vi "MirrorSlide2xPan.vi"(8 "error in (no error)":errorcluster caption="entrée d'erreur (pas d'erreur)", 11 "ESP301.lvclass":refnum<class "ESP301.lvclass">) -> (0 "error out":errorcluster caption="sortie d'erreur", 3 "ESP301.lvclass Out":refnum<class "ESP301.lvclass">)   [LabVIEW 2019, in "ESP301.lvclass"]
uses:
  ESP301.lvclass
  C:/Programmes Labview/LabScanV1A/DevicesClass/BaseDevice/BaseDevice.lvclass
  ESP301.lvclass/ESP301.ctl
  BaseDevice/ClassQueueMess.ctl
  BaseDevice/Accessor/GetClassEvent.vi
panel:
  out "ActPos 2":dbl=60.0 caption="Pos(mm)" min=0.1 step=0.1 format="%#.4f"
  in  "Motion ax2":u16(ring) caption="MiseAJour" items=["Cam", "APD", "Spectro"]
  out "Mvg_ax2":bool caption="Moving"
  out "Hmd_ax2":bool caption="Homed"
  in  "Axis 2":u8(ring)=1 items=["1"=1, "2"=2, "3"=3]
  in  "Con/Disc.":bool
  out "Hmd_ax1":bool caption="Homed"
  in  "Enable":bool
  in  "Home":bool caption="MiseAJour"
  out "Mvg_ax1":bool caption="Moving"
  out "Axis Model":string
  out "Valid Ref":bool
  out "BKD Lim":bool
  out "FWD Lim":bool
  in  "Axis 1":u8(ring)=1 items=["1"=1, "2"=2, "3"=3]
  out "ActPos":dbl=60.0 caption="Pos(mm)" min=0.1 step=0.1 format="%#.4f"
  in  "Target":dbl caption="Target(mm)" min=-25000.0 max=25000.0 step=0.0001 format="%#.4f"
  in  "Axis Name":string
  in  "MainProgQ":refnum<queue>
  in  "MainProgQEvent":refnum<user-event>
  in  "Acq":bool
  in  "Stop":bool
  in  "Motion ax1":u16(ring) caption="MiseAJour" items=["Cam", "APD", "Spectro"]
  out "Init Program":bool
  # "this MUST labeled with class name"
  # "this MUST be present and labeled \"Stop\" and \"Acq\""
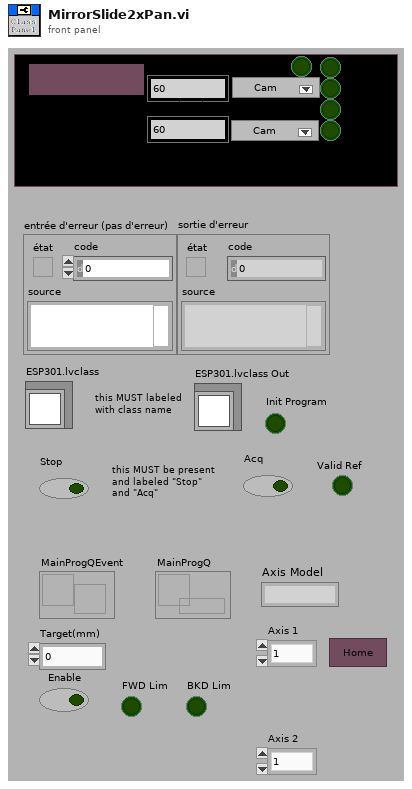
[diagram p1: front panel]
types:
  T1 = cluster{"ESP300mm":refnum<vi>, "ESP300ps":refnum<vi>, "MvgESP300":refnum<vi>}
  T2 = typedef "ClassQueueMess.ctl" = u16
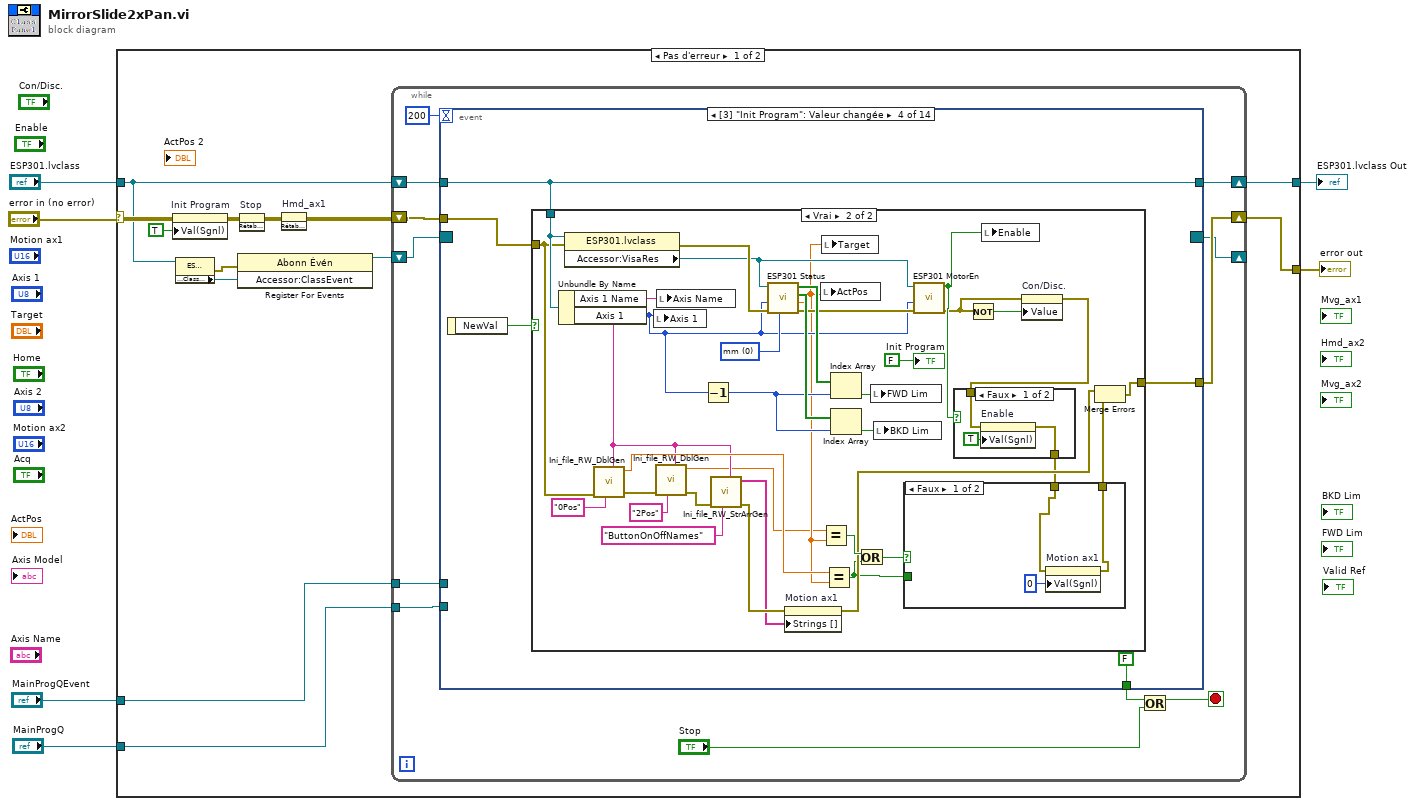
[diagram p0: block diagram]
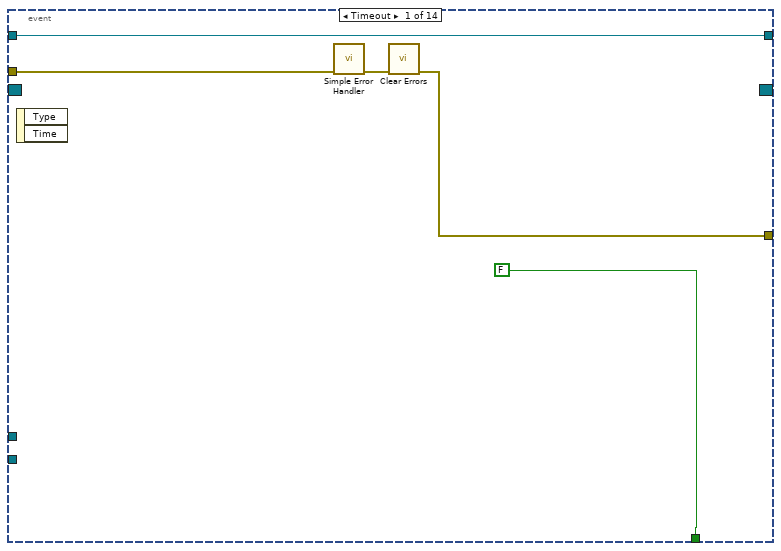
[diagram p2: hidden frame]
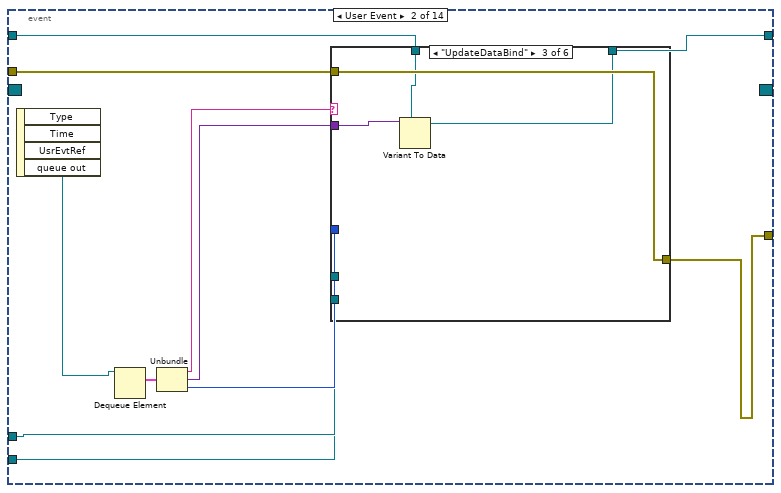
[diagram p3: hidden frame]
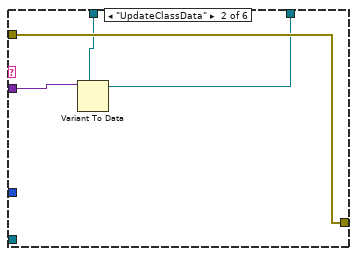
[diagram p5: hidden frame]
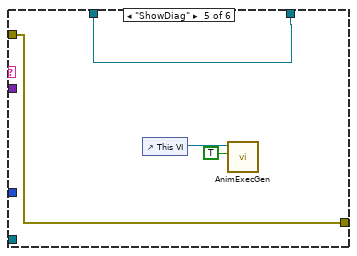
[diagram p7: hidden frame]
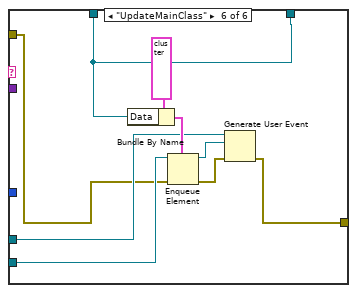
[diagram p8: hidden frame]
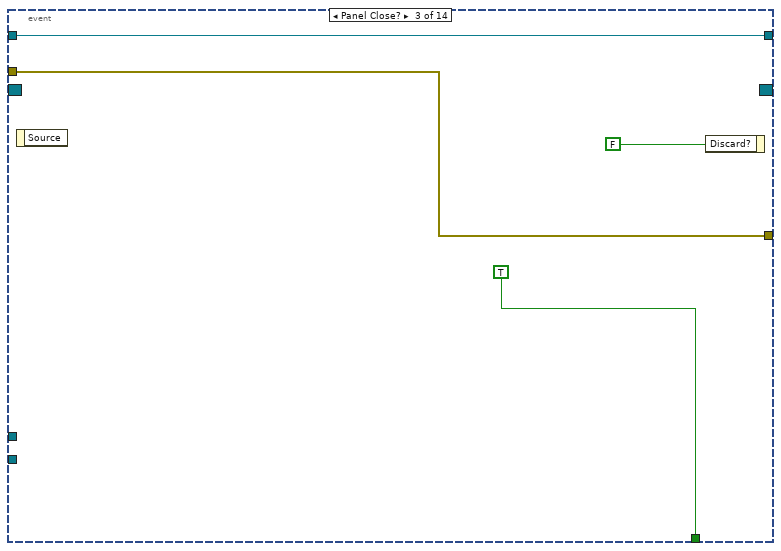
[diagram p9: hidden frame]
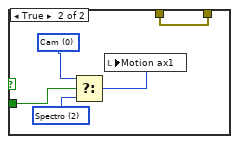
[diagram p12: hidden frame]
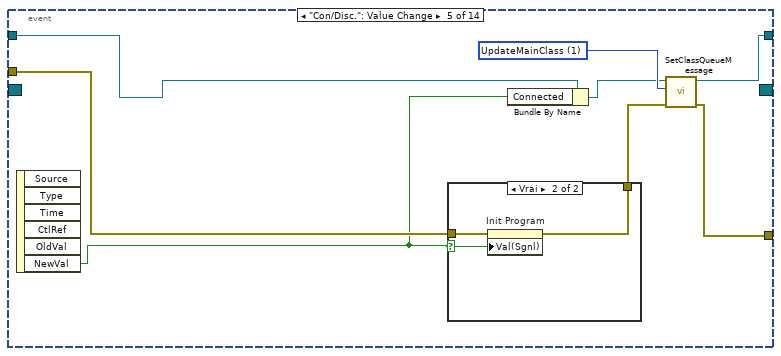
[diagram p13: hidden frame]
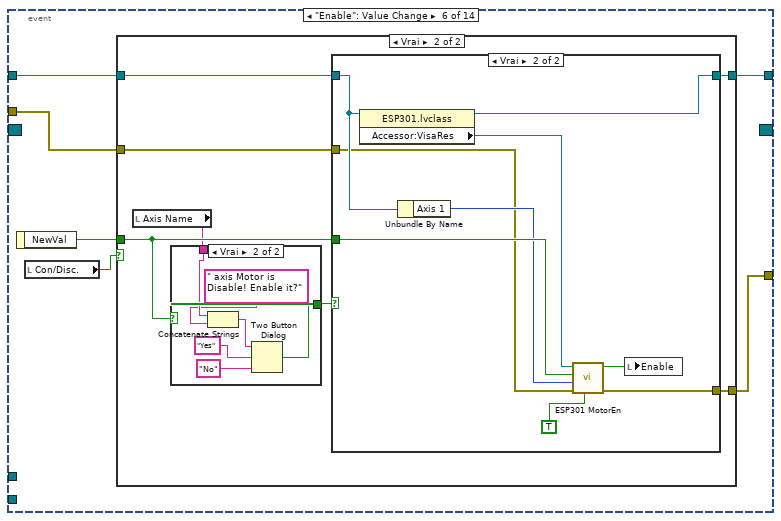
[diagram p15: hidden frame]
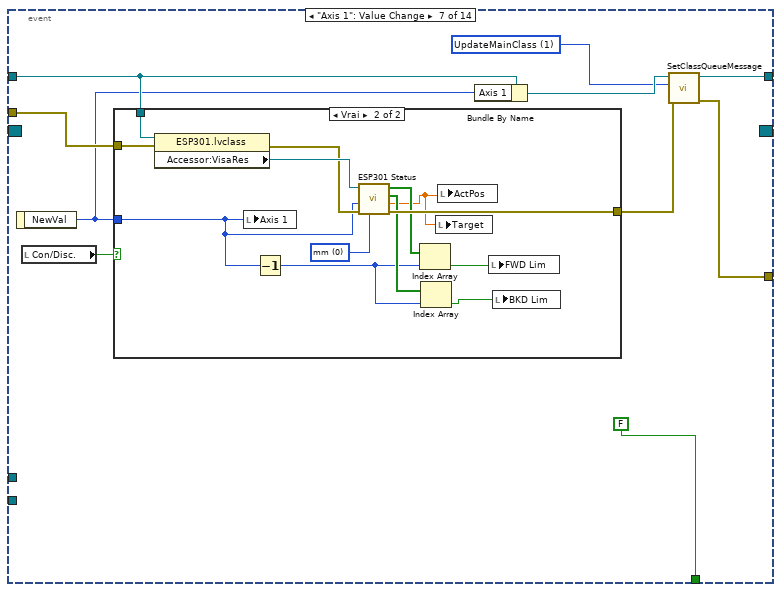
[diagram p19: hidden frame]
diagram:
  n1 = case shown="Pas d'erreur" "error in (no error)" {
    selector: "error in (no error)" -> [w16 w434]
    tunnel: [w19 w434] -> w5
    tunnel: "ESP301.lvclass" -> [w12 w433]
    tunnel: [w17 w433] -> w3
    tunnel: "MainProgQEvent" -> [w10 _]
    tunnel: "MainProgQ" -> [w9 _]
    frame No Error {
      n2 = property on="Init Program" class="Bool (strict)"(error in=w16, "Val(Sgnl)"=TRUE ("Valeur (Signalisation)")) -> (error out=w15:errorcluster)  [unwired: 1 in, 1 out]
      n3 = property class="ESP301.lvclass"(reference=w12) -> (error out=w14:errorcluster, "Accessor:ClassEvent"=w13:refnum<user-event>)  [unwired: 1 in, 1 out]
      n4 = register-events(error in=w14, w13) -> (reference out=w11:refnum<event-registration>)  [unwired: 1 in, 1 out]
      n5 = invoke on="Stop" class="Bool (strict)" method="RétablirValParDéfaut"(error in=w15) -> (error out=w8:errorcluster)  [unwired: 2 in, 2 out]
      n6 = invoke on="Hmd_ax1" class="Bool (strict)" method="RétablirValParDéfaut"(error in=w8) -> (error out=w7:errorcluster)  [unwired: 2 in, 2 out]
      n7 = while {
        shift-right: [w29] -> w19
        shift-left: w7 -> [w30]
        shift-right: [w27] -> w17
        shift-left: w12 -> [w28]
        shift-right: [w25] -> _
        shift-left: w11 -> [w26]
        tunnel: w10 -> [w24]
        tunnel: w9 -> [w23]
        stop <- w21 stop-if-true
        n8 = event shown="[3] \"Init Program\": Valeur changée" {
          selector: w26 -> [_ _ _ _ _ _ _ _ _ _ _ _ _ _]
          dyn-events: [_ _ _ _ _ _ _ _ _ _ _ _ _ _] -> w25
          timeout: 200 -> [_ _ _ _ _ _ _ _ _ _ _ _ _ _]
          tunnel: w30 -> [w34 w46 w74 w80 w133 w144 w184 w208 w226 w251 w294 w355 w369 w391]
          tunnel: [w32 w40 w74 w79 w130 w145 w179 w203 w225 w250 w292 w353 w368 w390] -> w29
          tunnel: w28 -> [w35 w47 w73 w77 w137 w146 w182 w206 w224 w249 w293 w354 w370 w392]
          tunnel: [FALSE _ TRUE FALSE _ _ FALSE FALSE _ _ _ _ _ _] -> w22
          tunnel: [w35 w39 w73 w77 w134 w147 w180 w204 w224 w249 w293 w354 w370 w393] -> w27
          tunnel: w24 -> [_ w38 _ _ _ _ _ _ _ _ _ _ _ _]
          tunnel: w23 -> [_ w37 _ _ _ _ _ _ _ _ _ _ _ _]
          event Timeout {
            n9 = event-data() -> ()  [unwired: 1 in, 2 out]
            n10 = call <vilib>:"Simple Error Handler.vi"("error in (no error)"=w34) -> ("error out"=w33:errorcluster)  [unwired: 4 in, 4 out]
            n11 = call <vilib>:"Clear Errors.vi"("error in (no error)"=w33) -> ("error out"=w32:errorcluster)  [unwired: 5 in, 1 out]
          }
          event User Event {
            n12 = event-data() -> ("queue out"=w44:refnum<queue>)  [unwired: 1 in, 3 out]
            n13 = Dequeue Element(queue=w44) -> (element=w45:cluster{"Message":string, "Data":variant, i32})  [unwired: 2 in, 3 out]
            n14 = Unbundle(w45) -> ("Message"=w43:string, "Data"=w42:variant, w41:i32)
            n15 = case shown="\"UpdateDataBind\"" w43 {
              tunnel: w46 -> [w49 w53 w57 w58 w62 w65]
              tunnel: w42 -> [_ w52 w56 _ _ _]
              tunnel: w47 -> [w48 w51 w55 w59 w63 w68]
              tunnel: [w48 w50 w54 w59 w63 w68] -> w39
              tunnel: [w49 w53 w57 w58 w62 w64] -> w40
              tunnel: w41 -> [_ _ _ _ _ _]
              tunnel: w38 -> [_ _ _ _ _ w67]
              tunnel: w37 -> [_ _ _ _ _ w66]
              frame Default {
              }
              frame "UpdateClassData" {
                n16 = Variant To Data(type=w51, Variant=w52) -> (data=w50:refnum<class "ESP301.lvclass">)  [unwired: 1 in, 1 out]
              }
              frame "UpdateDataBind" {
                n17 = Variant To Data(type=w55, Variant=w56) -> (data=w54:refnum<class "ESP301.lvclass">)  [unwired: 1 in, 1 out]
              }
              frame "MeasDone" {
              }
              frame "ShowDiag" {
                n18 = control-ref of="This VI"() -> (w61:refnum<vi>)
                n19 = call <userlib>:"AnimExecGen.vi"("Animer l'exécution ?"=TRUE, "ViRef"=w61) -> ()  [unwired: 9 in, 1 out]
              }
              frame "UpdateMainClass" {
                n20 = Bundle By Name(cluster=cluster{"Message":string, "Data":variant, i32} {"Message"="", "Data"=variant, 0} ("élément"), "Data"=w68) -> (w69:cluster{"Message":string, "Data":variant, i32})
                n21 = Enqueue Element(queue=w66, element=w69, error in (no error)=w65) -> (queue out=w72:refnum<queue>, error out=w71:errorcluster)  [unwired: 1 in, 1 out]
                n22 = Generate User Event(user event=w67, event data cluster=w72, error in=w71) -> (error out=w64:errorcluster)  [unwired: 1 in, 1 out]
              }
            }
          }
          event Panel Close? {
            n23 = event-data() -> ()  [unwired: 1 in, 1 out]
            n24 = event-data("Discard?"=FALSE ("Rejeter ?")) -> ()  [unwired: 1 in, 1 out]
          }
          event "Init Program": Value Change {
            n25 = event-data() -> ("NewVal"=w81:bool)  [unwired: 1 in]
            n26 = case shown="Vrai" w81 {
              tunnel: w80 -> [w82 w104]
              tunnel: [w82 w93] -> w79
              tunnel: w77 -> [_ w116]
              frame False {
              }
              frame True {
                w114 = i8 0 items=["mm", "ps"] ("Input Units")
                n27 = Unbundle By Name(w116) -> ("Axis 1 Name"=w96:string, "Axis 1"=w107:u8)
                n28 = property class="ESP301.lvclass"(reference=w116, error in=w104) -> (error out=w115:errorcluster, "Accessor:VisaRes"=w108:refnum<visa-resource-name>)  [unwired: 1 out]
                n29 = call <userlib>:"Ini_file_RW_DblGen.vi"("Section"=w96, "Key"="0Pos", "Error in"=w104) -> ("Error out"=w102:errorcluster, "ValueOut"=w101:dbl)  [unwired: 6 in]
                n30 = local write "Axis 1"(w107) -> ()
                n31 = call <userlib>:"Ini_file_RW_DblGen.vi"("Section"=w96, "Key"="2Pos", "Error in"=w102) -> ("Error out"=w97:errorcluster, "ValueOut"=w89:dbl)  [unwired: 6 in]
                n32 = local write "Axis Name"(w96) -> ()
                n33 = Decrement(x=w107) -> (x-1=w106:u8)
                n34 = call <userlib>:"Ini_file_RW_StrArrGen.vi"("Section"=w96, "Key"="ButtonOnOffNames", "Error in"=w97) -> ("Error out"=w94:errorcluster, "ValueOut"=w92:string[])  [unwired: 6 in]
                n35 = call <userlib>:"ESP301 Status.vi"("Input Units"=w114, "error in"=w115, "Axis"=w107, "VISA Rsrc"=w108) -> ("error out"=w109:errorcluster, "Position"=w100:dbl, "Low Limit"=w110:bool[], "High Limit"=w111:bool[])  [unwired: 4 in]
                n36 = property on="Motion ax1" class="MDér (strict)"(error in=w94, "Strings []"=w92) -> (error out=w91:errorcluster)  [unwired: 1 in, 1 out]
                n37 = local write "ActPos"(w100) -> ()
                n38 = Equal?(x=w89, y=w100) -> (x = y?=w99:bool)
                n39 = local write "Target"(w100) -> ()
                n40 = Equal?(x=w101, y=w100) -> (x = y?=w90:bool)
                n41 = Index Array(array=w111, index=w106) -> (element=w112:bool)
                n42 = Index Array(array=w110, index=w106) -> (element=w113:bool)
                n43 = Or(x=w99, y=w90) -> (x .or. y?=w98:bool)
                n44 = local write "FWD Lim"(w112) -> ()
                n45 = local write "BKD Lim"(w113) -> ()
                n46 = call <userlib>:"ESP301 MotorEn.vi"("error in"=w109, "Axis"=w107, "VISA Rsrc"=w108) -> ("error out"=w84:errorcluster, "MotorEnOut"=w88:bool)  [unwired: 7 in]
                n47 = Not(x=w84) -> (.not. x?=w85:bool)
                n48 = local write "Enable"(w88) -> ()
                n49 = property on="Con/Disc." class="Bool (strict)"(error in=w84, "Value"=w85) -> (error out=w83:errorcluster)  [unwired: 1 in, 1 out]
                n50 = case shown="Faux" w88 {
                  tunnel: w83 -> [w120 w121]
                  tunnel: [w119 w121] -> w87
                  frame False {
                    n51 = property on="Enable" class="Bool (strict)"(error in=w120, "Val(Sgnl)"=TRUE ("Valeur (Signalisation)")) -> (error out=w119:errorcluster)  [unwired: 1 in, 1 out]
                  }
                  frame True {
                  }
                }
                n52 = case shown="Faux" w98 {
                  tunnel: w90 -> [_ w129]
                  tunnel: w87 -> [w122 w125]
                  tunnel: [w123 w125] -> w86
                  frame False {
                    n53 = property on="Motion ax1" class="MDér (strict)"(error in=w122, "Val(Sgnl)"=u16 0 ("Valeur (Signalisation)")) -> (error out=w123:errorcluster)  [unwired: 1 in, 1 out]
                  }
                  frame True {
                    w128 = u16 2 items=["Cam", "APD", "Spectro"] ("MirrorMotion")
                    w127 = u16 0 items=["Cam", "APD", "Spectro"] ("MirrorMotion")
                    n54 = Select(t=w127, s=w129, f=w128) -> (s? t:f=w126:u16)
                    n55 = local write "Motion ax1"(w126) -> ()
                  }
                }
                n56 = Merge Errors(w91, w86) -> (w93:errorcluster)
                "Init Program" <- FALSE
              }
            }
          }
          event "Con/Disc.": Value Change {
            w136 = T2 1 items=["UpdateClassData", "UpdateMainClass", "UpdateDataBind", "ReInitDevice", "Custom", "ClosePan"] ("Menu déroulant")
            n57 = event-data() -> ("NewVal"=w132:bool)  [unwired: 1 in, 5 out]
            n58 = case shown="Vrai" w132 {
              selector: w132 -> [_ w140]
              tunnel: w133 -> [w138 w141]
              tunnel: [w138 w139] -> w131
              frame False {
              }
              frame True {
                n59 = property on="Init Program" class="Bool (strict)"(error in=w141, "Val(Sgnl)"=w140) -> (error out=w139:errorcluster)  [unwired: 1 in, 1 out]
              }
            }
            n60 = Bundle By Name(cluster=w137, "Connected"=w132) -> (w135:refnum<class "ESP301.lvclass">)
            n61 = call-dynamic "SetClassQueueMessage.vi"("ErrorIn(No Error)"=w131, "Menu déroulant"=w136, "DefaultDev.lvclass"=w135) -> ("sortie d'erreur"=w130:errorcluster, "DefaultDev.lvclass Out"=w134:refnum<class "ESP301.lvclass">)  [unwired: 7 in]
          }
          event "Enable": Value Change {
            n62 = event-data() -> ("NewVal"=w143:bool)  [unwired: 1 in]
            n63 = local read "Con/Disc."() -> (w142:bool)
            n64 = case shown="Vrai" w142 {
              tunnel: [w149 w156] -> w147
              tunnel: w146 -> [w149 w155]
              tunnel: [w148 w154] -> w145
              tunnel: w144 -> [w148 w153]
              tunnel: w143 -> [_ w151]
              frame False {
              }
              frame True {
                n65 = local read "Axis Name"() -> (w150:string)
                n66 = case shown="Vrai" w151 {
                  selector: w151 -> [w157 _]
                  tunnel: [w157 w161] -> w152
                  tunnel: w150 -> [_ w160]
                  frame False {
                  }
                  frame True {
                    n67 = Concatenate Strings(w160, " axis Motor is Disable! Enable it?" ("message")) -> (w158:string)
                    n68 = Two Button Dialog(message=w158, 1:"No" ("Nom du bouton F (\"Annuler\")"), 2:"Yes" ("Nom du bouton V (\"OK\")")) -> (T button?=w161:bool)
                  }
                }
                n69 = case shown="Vrai" w152 {
                  tunnel: w151 -> [_ w171]
                  tunnel: [w164 w170] -> w156
                  tunnel: w155 -> [w164 w169]
                  tunnel: [w165 w167] -> w154
                  tunnel: w153 -> [w165 w166]
                  frame False {
                  }
                  frame True {
                    n70 = property class="ESP301.lvclass"(reference=w169) -> (reference out=w170:refnum<class "ESP301.lvclass">, "Accessor:VisaRes"=w173:refnum<visa-resource-name>)  [unwired: 1 in, 1 out]
                    n71 = Unbundle By Name(w169) -> ("Axis 1"=w168:u8)
                    n72 = call <userlib>:"ESP301 MotorEn.vi"("Set"=TRUE, "error in"=w166, "Axis"=w168, "MotorEn"=w171, "VISA Rsrc"=w173) -> ("error out"=w167:errorcluster, "MotorEnOut"=w174:bool)  [unwired: 5 in]
                    n73 = local write "Enable"(w174) -> ()
                  }
                }
              }
            }
          }
          event "Axis 1": Value Change {
            w178 = T2 1 items=["UpdateClassData", "UpdateMainClass", "UpdateDataBind", "ReInitDevice", "Custom", "ClosePan"] ("Menu déroulant")
            n74 = event-data() -> ("NewVal"=w175:u8)  [unwired: 1 in]
            n75 = local read "Con/Disc."() -> (w176:bool)
            n76 = case shown="Vrai" w176 {
              tunnel: w184 -> [w185 w198]
              tunnel: w182 -> [_ w197]
              tunnel: [w185 w194] -> w177
              tunnel: w175 -> [_ w188]
              frame False {
              }
              frame True {
                w193 = i8 0 items=["mm", "ps"] ("Input Units")
                n77 = property class="ESP301.lvclass"(reference=w197, error in=w198) -> (error out=w195:errorcluster, "Accessor:VisaRes"=w196:refnum<visa-resource-name>)  [unwired: 1 out]
                n78 = local write "Axis 1"(w188) -> ()
                n79 = Decrement(x=w188) -> (x-1=w187:u8)
                n80 = call <userlib>:"ESP301 Status.vi"("Input Units"=w193, "error in"=w195, "Axis"=w188, "VISA Rsrc"=w196) -> ("error out"=w194:errorcluster, "Position"=w186:dbl, "Low Limit"=w189:bool[], "High Limit"=w192:bool[])  [unwired: 4 in]
                n81 = Index Array(array=w192, index=w187) -> (element=w190:bool)
                n82 = Index Array(array=w189, index=w187) -> (element=w191:bool)
                n83 = local write "Target"(w186) -> ()
                n84 = local write "ActPos"(w186) -> ()
                n85 = local write "FWD Lim"(w190) -> ()
                n86 = local write "BKD Lim"(w191) -> ()
              }
            }
            n87 = Bundle By Name(cluster=w182, "Axis 1"=w175) -> (w181:refnum<class "ESP301.lvclass">)
            n88 = call-dynamic "SetClassQueueMessage.vi"("ErrorIn(No Error)"=w177, "Menu déroulant"=w178, "DefaultDev.lvclass"=w181) -> ("sortie d'erreur"=w179:errorcluster, "DefaultDev.lvclass Out"=w180:refnum<class "ESP301.lvclass">)  [unwired: 7 in]
          }
          event "Axis 2": Value Change {
            w202 = T2 1 items=["UpdateClassData", "UpdateMainClass", "UpdateDataBind", "ReInitDevice", "Custom", "ClosePan"] ("Menu déroulant")
            n89 = event-data() -> ("NewVal"=w199:u8)  [unwired: 1 in]
            n90 = local read "Con/Disc."() -> (w200:bool)
            n91 = case shown="Vrai" w200 {
              tunnel: w208 -> [w209 w222]
              tunnel: w206 -> [_ w221]
              tunnel: [w209 w218] -> w201
              tunnel: w199 -> [_ w212]
              frame False {
              }
              frame True {
                w217 = i8 0 items=["mm", "ps"] ("Input Units")
                n92 = property class="ESP301.lvclass"(reference=w221, error in=w222) -> (error out=w219:errorcluster, "Accessor:VisaRes"=w220:refnum<visa-resource-name>)  [unwired: 1 out]
                n93 = local write "Axis 2"(w212) -> ()
                n94 = Decrement(x=w212) -> (x-1=w211:u8)
                n95 = call <userlib>:"ESP301 Status.vi"("Input Units"=w217, "error in"=w219, "Axis"=w212, "VISA Rsrc"=w220) -> ("error out"=w218:errorcluster, "Position"=w210:dbl, "Low Limit"=w213:bool[], "High Limit"=w216:bool[])  [unwired: 4 in]
                n96 = Index Array(array=w216, index=w211) -> (element=w214:bool)
                n97 = Index Array(array=w213, index=w211) -> (element=w215:bool)
                n98 = local write "Target"(w210) -> ()
                n99 = local write "ActPos"(w210) -> ()
                n100 = local write "FWD Lim"(w214) -> ()
                n101 = local write "BKD Lim"(w215) -> ()
              }
            }
            n102 = Bundle By Name(cluster=w206, "Axis 2"=w199) -> (w205:refnum<class "ESP301.lvclass">)
            n103 = call-dynamic "SetClassQueueMessage.vi"("ErrorIn(No Error)"=w201, "Menu déroulant"=w202, "DefaultDev.lvclass"=w205) -> ("sortie d'erreur"=w203:errorcluster, "DefaultDev.lvclass Out"=w204:refnum<class "ESP301.lvclass">)  [unwired: 7 in]
          }
          event "Home": Value Change {
            n104 = event-data() -> ("NewVal"=w227:bool)  [unwired: 1 in]
            n105 = local read "Con/Disc."() -> (w223:bool)
            n106 = case shown="Vrai" w223 {
              tunnel: w227 -> [_ w232]
              tunnel: w224 -> [_ w231]
              tunnel: w226 -> [w228 w230]
              tunnel: [w228 w229] -> w225
              frame False {
              }
              frame True {
                n107 = case shown="Vrai" w232 {
                  tunnel: w231 -> [_ w247]
                  tunnel: w230 -> [w233 w239]
                  tunnel: [w233 w237] -> w229
                  frame False {
                  }
                  frame True {
                    w243 = i8 0 items=["mm", "ps"] ("Input Units")
                    n108 = property class="ESP301.lvclass"(reference=w247, error in=w239) -> (error out=w245:errorcluster, "Accessor:VisaRes"=w246:refnum<visa-resource-name>)  [unwired: 1 out]
                    n109 = control-ref of="Mvg_ax1"() -> (w238:refnum<vi>)
                    n110 = control-ref of="ActPos"() -> (w241:refnum<vi>)
                    n111 = local read "Axis 1"() -> (w244:u8)
                    n112 = Bundle By Name(cluster=T1 {"ESP300mm"=refnum, "ESP300ps"=refnum, "MvgESP300"=refnum} ("ESP301Ref"), "ESP300mm"=w241, "MvgESP300"=w238) -> (w240:T1)
                    n113 = call <userlib>:"ESP301 Home.vi"("Input Units"=w243, "ESP301Ref"=w240, "error in"=w245, "Axis"=w244, "VISA Rsrc"=w246) -> ("error out"=w237:errorcluster)  [unwired: 6 in]
                    n114 = call <userlib>:"Wait_At_Wire_Bool.vi"("Wait (ms)"=u32 250, "error in (no error)"=FALSE) -> ("error out"=w236:bool)  [unwired: 7 in, 2 out]
                    n115 = local write "Home"(w236) -> ()
                  }
                }
              }
            }
          }
          event "Motion ax1": Value Change {
            n116 = event-data() -> ("NewVal"=w252:u16)  [unwired: 1 in]
            n117 = local read "Con/Disc."() -> (w248:bool)
            n118 = case shown="Vrai" w248 {
              tunnel: w252 -> [_ w258]
              tunnel: w251 -> [w253 w257]
              tunnel: [w253 w256] -> w250
              tunnel: w249 -> [_ w254]
              frame False {
              }
              frame True {
                n119 = local read "Axis Name"() -> (w255:string)
                n120 = case shown="0, Par défaut" w258 {
                  tunnel: w257 -> [w267 w282 w288]
                  tunnel: [w261 w284 w290] -> w256
                  tunnel: w254 -> [w266 _ _]
                  tunnel: w255 -> [w259 w279 w285]
                  frame 0, Default {
                    w268 = i8 0 items=["mm", "ps"] ("Input Units")
                    # "Cam"
                    n121 = property class="ESP301.lvclass"(reference=w266, error in=w267) -> (error out=w277:errorcluster, "Accessor:VisaRes"=w278:refnum<visa-resource-name>)  [unwired: 1 out]
                    n122 = control-ref of="Mvg_ax1"() -> (w273:refnum<vi>)
                    n123 = control-ref of="ActPos"() -> (w275:refnum<vi>)
                    n124 = local read "Axis 1"() -> (w276:u8)
                    n125 = Bundle By Name(cluster=T1 {"ESP300mm"=refnum, "ESP300ps"=refnum, "MvgESP300"=refnum} ("ESP301Ref"), "ESP300mm"=w275, "MvgESP300"=w273) -> (w274:T1)
                    n126 = call <userlib>:"ESP301 Home.vi"("Input Units"=w268, "ESP301Ref"=w274, "error in"=w277, "Axis"=w276, "VISA Rsrc"=w278) -> ("error out"=w264:errorcluster)  [unwired: 6 in]
                    n127 = call <userlib>:"Wait_At_Wire_Bool.vi"("Wait (ms)"=u32 250, "error in (no error)"=FALSE) -> ("error out"=w272:bool)  [unwired: 7 in, 2 out]
                    n128 = call <userlib>:"Ini_file_RW_DblGen.vi"("Section"=w259, "Key"="0Pos", "Error in"=w264) -> ("Error out"=w263:errorcluster, "ValueOut"=w262:dbl)  [unwired: 6 in]
                    n129 = local write "Home"(w272) -> ()
                    n130 = property on="Target" class="NumNb (strict)"(error in=w263, "Val(Sgnl)"=w262) -> (error out=w261:errorcluster)  [unwired: 1 in, 1 out]
                    "Hmd_ax1" <- TRUE ("Homed")
                  }
                  frame 1 {
                    # "APD"
                    n131 = call <userlib>:"Ini_file_RW_DblGen.vi"("Section"=w279, "Key"="1Pos", "Error in"=w282) -> ("Error out"=w281:errorcluster, "ValueOut"=w283:dbl)  [unwired: 6 in]
                    n132 = property on="Target" class="NumNb (strict)"(error in=w281, "Val(Sgnl)"=w283) -> (error out=w284:errorcluster)  [unwired: 1 in, 1 out]
                  }
                  frame 2 {
                    # "Spectro"
                    n133 = call <userlib>:"Ini_file_RW_DblGen.vi"("Section"=w285, "Key"="2Pos", "Error in"=w288) -> ("Error out"=w287:errorcluster, "ValueOut"=w289:dbl)  [unwired: 6 in]
                    n134 = property on="Target" class="NumNb (strict)"(error in=w287, "Val(Sgnl)"=w289) -> (error out=w290:errorcluster)  [unwired: 1 in, 1 out]
                  }
                }
              }
            }
          }
          event "Motion ax1": Shortcut Menu Selection (User) {
            n135 = event-data() -> ("ItemTag"=w295:string)  [unwired: 1 in]
            n136 = local read "Axis Name"() -> (w291:string)
            n137 = case shown="\"ElementsNames\"" w295 {
              tunnel: w294 -> [w296 w302 w316 w331 w343]
              tunnel: [w296 w304 w319 w330 w342] -> w292
              tunnel: w291 -> [_ w303 w317 w328 w340]
              frame Default {
              }
              frame "ElementsNames" {
                n138 = call "Set Button Elements Text"("error in (no error)"=w302) -> ("Button 2 Text"=w297:string, "Button 1 Text"=w298:string, "Button 0 Text"=w299:string, "Save"=w300:bool, "error out"=w301:errorcluster)  [unwired: 14 in]
                n139 = case shown="Vrai" w300 {
                  tunnel: w301 -> [w305 w312]
                  tunnel: [w305 w311] -> w304
                  tunnel: w303 -> [_ w310]
                  tunnel: w299 -> [_ w309]
                  tunnel: w298 -> [_ w308]
                  tunnel: w297 -> [_ w306]
                  frame False {
                  }
                  frame True {
                    n140 = Build Array(w309, w308, w306) -> (w307:string[])
                    n141 = property on="Motion ax1" class="MDér (strict)"("Strings []"=w307) -> ()  [unwired: 2 in, 2 out]
                    n142 = call <userlib>:"Ini_file_RW_StrArrGen.vi"("Section"=w310, "Key"="ButtonOnOffNames", "Error in"=w312, "Write"=TRUE, "ValueIn"=w307) -> ("Error out"=w311:errorcluster)  [unwired: 4 in, 1 out]
                  }
                }
              }
              frame "0 Position" {
                n143 = call "Set Element 0 Position"("error in (no error)"=w316) -> ("Element 0 Position(mm)"=w320:dbl, "Save"=w318:bool, "error out"=w315:errorcluster)  [unwired: 16 in]
                n144 = case shown="Vrai" w318 {
                  tunnel: w320 -> [_ w327]
                  tunnel: w315 -> [w321 w324]
                  tunnel: [w321 w323] -> w319
                  tunnel: w317 -> [_ w322]
                  frame False {
                  }
                  frame True {
                    n145 = call <userlib>:"Ini_file_RW_DblGen.vi"("Section"=w322, "Key"="0Pos", "Error in"=w324, "Write"=TRUE, "ValueIn"=w327) -> ("Error out"=w323:errorcluster)  [unwired: 4 in, 1 out]
                  }
                }
              }
              frame "1 Position" {
                n146 = call "Set Element 1 Position"() -> ("Element 1 Position(mm)"=w332:dbl, "Save"=w329:bool)  [unwired: 17 in, 1 out]
                n147 = case shown="Vrai" w329 {
                  tunnel: w332 -> [_ w339]
                  tunnel: w331 -> [w333 w336]
                  tunnel: [w333 w335] -> w330
                  tunnel: w328 -> [_ w334]
                  frame False {
                  }
                  frame True {
                    n148 = call <userlib>:"Ini_file_RW_DblGen.vi"("Section"=w334, "Key"="1Pos", "Error in"=w336, "Write"=TRUE, "ValueIn"=w339) -> ("Error out"=w335:errorcluster)  [unwired: 4 in, 1 out]
                  }
                }
              }
              frame "2 Position" {
                n149 = call "Set Element 2 Position"() -> ("Element 2 Position(mm)"=w344:dbl, "Save"=w341:bool)  [unwired: 17 in, 1 out]
                n150 = case shown="Vrai" w341 {
                  tunnel: w344 -> [_ w351]
                  tunnel: w343 -> [w345 w348]
                  tunnel: [w345 w347] -> w342
                  tunnel: w340 -> [_ w346]
                  frame False {
                  }
                  frame True {
                    n151 = call <userlib>:"Ini_file_RW_DblGen.vi"("Section"=w346, "Key"="2Pos", "Error in"=w348, "Write"=TRUE, "ValueIn"=w351) -> ("Error out"=w347:errorcluster)  [unwired: 4 in, 1 out]
                  }
                }
              }
            }
          }
          event "ActPos": Shortcut Menu Selection (User) {
            n152 = event-data() -> ("ItemTag"=w356:string)  [unwired: 1 in]
            n153 = local read "Axis Name"() -> (w352:string)
            n154 = case shown="\"Goto\"" w356 {
              tunnel: w355 -> [w357 w361]
              tunnel: [w357 w360] -> w353
              tunnel: w352 -> [_ w358]
              frame Default {
              }
              frame "Goto" {
                n155 = call "Go to Position"() -> ("Target Position(mm)"=w362:dbl, "Goto"=w359:bool)  [unwired: 17 in, 1 out]
                n156 = case shown="Vrai" w359 {
                  tunnel: w362 -> [_ w364]
                  tunnel: w361 -> [w363 w365]
                  tunnel: [w363 w365] -> w360
                  tunnel: w358 -> [_ _]
                  frame False {
                  }
                  frame True {
                    n157 = property on="Target" class="NumNb (strict)"("Val(Sgnl)"=w364) -> ()  [unwired: 2 in, 2 out]
                  }
                }
              }
            }
          }
          event "Target": Value Change {
            n158 = event-data() -> ("NewVal"=w367:dbl)  [unwired: 1 in]
            n159 = local read "Con/Disc."() -> (w366:bool)
            n160 = case shown="Vrai" w366 {
              tunnel: w370 -> [_ w387]
              tunnel: w369 -> [w371 w386]
              tunnel: [w371 w379] -> w368
              tunnel: w367 -> [_ w378]
              frame False {
              }
              frame True {
                w380 = i8 0 items=["mm", "ps"] ("Input Units")
                n161 = property class="ESP301.lvclass"(reference=w387, error in=w386) -> (error out=w382:errorcluster, "Accessor:VisaRes"=w383:refnum<visa-resource-name>)  [unwired: 1 out]
                n162 = control-ref of="Mvg_ax1"() -> (w384:refnum<vi>)
                n163 = control-ref of="ActPos"() -> (w385:refnum<vi>)
                n164 = local read "Axis 1"() -> (w381:u8)
                n165 = Bundle By Name(cluster=T1 {"ESP300mm"=refnum, "ESP300ps"=refnum, "MvgESP300"=refnum} ("ESP301Ref"), "ESP300mm"=w385, "MvgESP300"=w384) -> (w373:T1)
                n166 = call <userlib>:"ESP301 Goto.vi"("Input Units"=w380, "ESP301Ref"=w373, "error in"=w382, "Axis"=w381, "Position"=w378, "VISA Rsrc"=w383) -> ("error out"=w379:errorcluster, "HighLim"=w375:bool, "Pos Out"=w377:dbl, "Warning"=w374:bool, "LowLim"=w376:bool)  [unwired: 1 in]
                n167 = local write "ActPos"(w377) -> ()
                n168 = case shown="Vrai" w374 {
                  tunnel: w376 -> [_ w389]
                  tunnel: w375 -> [_ w388]
                  frame False {
                  }
                  frame True {
                    n169 = local write "FWD Lim"(w388) -> ()
                    n170 = local write "BKD Lim"(w389) -> ()
                  }
                }
              }
            }
          }
          event "Axis Name": Shortcut Menu Selection (User) {
            n171 = event-data() -> ("ItemTag"=w394:string)  [unwired: 1 in]
            n172 = case shown="\"ChangeName\"" w394 {
              tunnel: [w396 w400 w411 w415 w420] -> w393
              tunnel: w392 -> [w396 w400 w411 w415 w421]
              tunnel: w391 -> [w395 w399 w409 w413 w422]
              tunnel: [w395 w397 w408 w412 w417] -> w390
              frame Default {
              }
              frame "Change Axis" {
                n173 = call "Set Mirror Axis"("error in (no error)"=w399) -> ("Mirror Axis"=w402:dbl, "Save"=w401:bool, "error out"=w398:errorcluster)  [unwired: 16 in]
                n174 = case shown="Vrai" w401 {
                  tunnel: w398 -> [w403 w407]
                  tunnel: [w403 w406] -> w397
                  tunnel: w402 -> [_ w405]
                  frame False {
                  }
                  frame True {
                    n175 = To Unsigned Byte Integer(number=w405) -> (unsigned 8bit integer=w404:u8)
                    n176 = property on="Axis 1" class="MDér (strict)"(error in=w407, "Val(Sgnl)"=w404) -> (error out=w406:errorcluster)  [unwired: 1 in, 1 out]
                  }
                }
              }
              frame "Home Axis" {
                n177 = property on="Home" class="Bool (strict)"(error in=w409, "Val(Sgnl)"=TRUE ("Valeur (Signalisation)")) -> (error out=w408:errorcluster)  [unwired: 1 in, 1 out]
              }
              frame "EnableAxis" {
                n178 = property on="Enable" class="Bool (strict)"(error in=w413, "Val(Sgnl)"=TRUE ("Valeur (Signalisation)")) -> (error out=w412:errorcluster)  [unwired: 1 in, 1 out]
              }
              frame "ChangeName" {
                n179 = call "SaveAxisName"("Enable"=TRUE, "error in (no error)"=w422) -> ("Name"=w416:string, "Save"=w419:bool, "error out"=w418:errorcluster)  [unwired: 15 in]
                n180 = case shown="Vrai" w419 {
                  tunnel: w421 -> [w425 w432]
                  tunnel: [w425 w430] -> w420
                  tunnel: w418 -> [w424 w429]
                  tunnel: [w424 w428] -> w417
                  tunnel: w416 -> [_ w427]
                  frame False {
                  }
                  frame True {
                    w426 = T2 1 items=["UpdateClassData", "UpdateMainClass", "UpdateDataBind", "ReInitDevice", "Custom", "ClosePan"] ("Menu déroulant")
                    n181 = Bundle By Name(cluster=w432, "Axis 1 Name"=w427) -> (w431:refnum<class "ESP301.lvclass">)
                    n182 = local write "Axis Name"(w427) -> ()
                    n183 = call-dynamic "SetClassQueueMessage.vi"("ErrorIn(No Error)"=w429, "Menu déroulant"=w426, "DefaultDev.lvclass"=w431) -> ("sortie d'erreur"=w428:errorcluster, "DefaultDev.lvclass Out"=w430:refnum<class "ESP301.lvclass">)  [unwired: 7 in]
                  }
                }
              }
            }
          }
        }
        n184 = Or(x=w22, y="Stop") -> (x .or. y?=w21:bool)
      }
    }
    frame Error {
    }
  }
  "error out" <- w5
  "ESP301.lvclass Out" <- w3
